vi "HowToAdjustAngle.vi"(11 "Current Sailing Regime":T1) -> (3 "Desired Sailing Regime":T1)   [LabVIEW 2013]
doc: "This VI is only called when we are in the correct regime and we want to make an angle change within the regime to our desired heading, and it determines which transition the boat should use to adjust the heading of the boat to the desired heading.\n\nPassing Transition regimes into this VI will break it. Nothin will crash, but the output will be meaningless - a steady-state regime (e.g. Upwind - Starboard Tack) will be the output.\n\nEric Schneider, Feb. 2014"
uses:
  Data/TypeDefs/Sailing Regimes.ctl
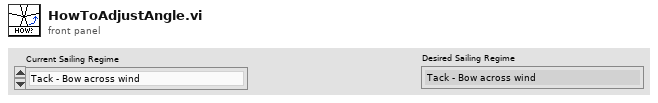
[diagram p1: front panel]
types:
  T1 = typedef "Sailing Regimes.ctl" = enum16{"Tack - Bow across wind", "Upwind - Starboard Tack", "Turn between Upwind/Reach - Starboard Tack", "Reach - Starboard Tack", "Turn between Reach/Run - Starboard Tack", "Run - Starboard Tack", "Jibe - Stern across wind", "Run - Port Tack", "Turn between Reach/Run - Port Tack", "Reach - Port Tack", "Turn between Upwind/Reach - Port Tack", "Upwind - Port Tack"}
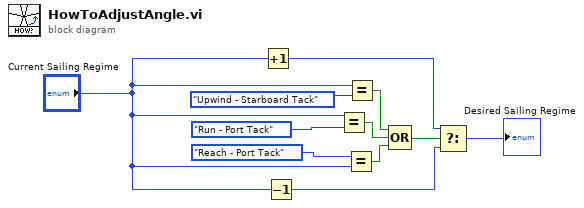
[diagram p0: block diagram]
diagram:
  n1 = Increment(x="Current Sailing Regime") -> (x+1=w5:T1)
  n2 = Decrement(x="Current Sailing Regime") -> (x-1=w4:T1)
  n3 = Equal?(x="Current Sailing Regime", y=Sailing_Regimes."Run - Port Tack") -> (x = y?=w8:bool)
  n4 = Equal?(x=Sailing_Regimes."Reach - Port Tack" ("y"), y="Current Sailing Regime") -> (x = y?=w9:bool)
  n5 = Equal?(x="Current Sailing Regime", y=Sailing_Regimes."Upwind - Starboard Tack") -> (x = y?=w7:bool)
  n6 = Compound Arithmetic op=OR(w7, w8, w9) -> (w6:bool)
  n7 = Select(t=w5, s=w6, f=w4) -> (s? t:f=→"Desired Sailing Regime":T1)
